vi "S4ACS_Controller.vi"() -> ()   [LabVIEW 2018]
uses:
  Channel Manager/Channel Manager.lvclass
  Channel/Channel.lvclass
panel:
  in  "Stop Button":bool
  in  "Camera ID":u8=1
  in  "Channel Manager.lvclass":refnum<class "Channel Manager.lvclass">
  out "GUI Message":string
  out "Error":string
  # "Welcome to the\nAcquisition Control System (ACS)\nof the SPARC4 instrument"
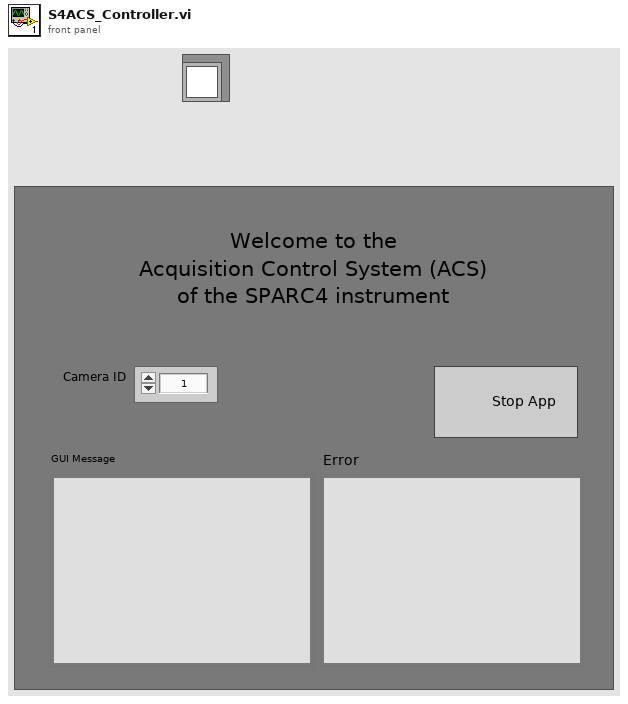
[diagram p1: front panel]
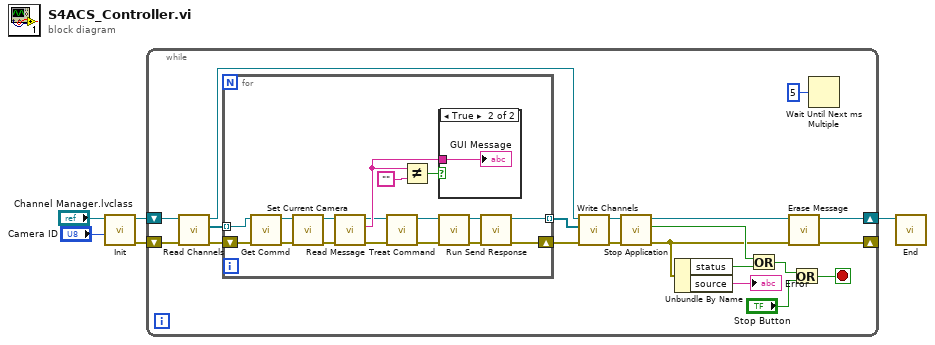
[diagram p0: block diagram]
diagram:
  n1 = call "Init.vi"("Computer Specifier"="Camera ID", "Channel Manager in"="Channel Manager.lvclass") -> ("error out"=w4:errorcluster, "Channel Manager out"=w5:refnum<class "Channel Manager.lvclass">)  [unwired: 8 in]
  n2 = while {
    shift-right: [w7] -> _
    shift-left: w4 -> [w9]
    shift-right: [w8] -> w3
    shift-left: w5 -> [w10]
    stop <- w11 stop-if-true
    n3 = call "Read Channels.vi"("error in (no error)"=w9, "Channel Manager in"=w10) -> ("error out"=w24:errorcluster, "Array"=w25:refnum<class "Channel.lvclass">[], "Channel Manager out"=w22:refnum<class "Channel Manager.lvclass">)  [unwired: 7 in]
    n4 = for {
      tunnel: w25 -> [w36] mode=indexing
      tunnel: [w26] -> w23 mode=indexing
      shift-right: [w27] -> w21
      shift-left: w24 -> [w37]
      n5 = call "Get Commd.vi"("error in (no error)"=w37, "Channel in"=w36) -> ("error out"=w30:errorcluster, "Channel out"=w31:refnum<class "Channel.lvclass">)  [unwired: 8 in]
      n6 = call "Set Current Camera.vi"("error in (no error)"=w30, "Channel in"=w31) -> ("error out"=w39:errorcluster, "Channel out"=w38:refnum<class "Channel.lvclass">)  [unwired: 8 in]
      n7 = call "Read Message.vi"("error in (no error)"=w39, "Channel in"=w38) -> ("error out"=w33:errorcluster, "Message"=w40:string, "Channel out"=w34:refnum<class "Channel.lvclass">)  [unwired: 7 in]
      n8 = call "Treat Command.vi"("error in (no error)"=w33, "Channel in"=w34) -> ("error out"=w32:errorcluster, "Channel out"=w35:refnum<class "Channel.lvclass">)  [unwired: 8 in]
      n9 = Not Equal?(x=w40, y="") -> (x != y?=w41:bool)
      n10 = case shown="True" w41 {
        tunnel: w40 -> [_ w43]
        frame False {
        }
        frame True {
          "GUI Message" <- w43
        }
      }
      n11 = call "Run.vi"("error in (no error)"=w32, "Channel in"=w35) -> ("error out"=w28:errorcluster, "Channel out"=w29:refnum<class "Channel.lvclass">)  [unwired: 8 in]
      n12 = call "Send Response.vi"("error in (no error)"=w28, "Channel in"=w29) -> ("error out"=w27:errorcluster, "Channel out"=w26:refnum<class "Channel.lvclass">)  [unwired: 8 in]
    }
    n13 = call "Write Channels.vi"("error in (no error)"=w21, "Channels Array"=w23, "Channel Manager in"=w22) -> ("error out"=w20:errorcluster, "Channel Manager out"=w19:refnum<class "Channel Manager.lvclass">)  [unwired: 7 in]
    n14 = call "Stop Application.vi"("error in (no error)"=w20, "Channel Manager in"=w19) -> ("error out"=w16:errorcluster, "Stop Application"=w17:bool, "Channel Manager out"=w15:refnum<class "Channel Manager.lvclass">)  [unwired: 7 in]
    n15 = Unbundle By Name(w16) -> ("status"=w18:bool, "source"=→"Error":string)
    n16 = Or(x=w17, y=w18) -> (x .or. y?=w13:bool)
    n17 = call "Erase Message.vi"("error in (no error)"=w16, "Channel Manager in"=w15) -> ("error out"=w7:errorcluster, "Channel Manager out"=w8:refnum<class "Channel Manager.lvclass">)  [unwired: 8 in]
    n18 = Or(x=w13, y="Stop Button") -> (x .or. y?=w11:bool)
    n19 = Wait Until Next ms Multiple(millisecond multiple=u32 5) -> ()  [unwired: 1 out]
  }
  n20 = call "End.vi"("Channel Manager in"=w3) -> ()  [unwired: 9 in, 2 out]
